vi "test_riccat_01i.vi"() -> (3 "All Tests Passed":bool)   [LabVIEW 2019]
uses:
  <vilib>/Analysis/Matrix/Datatypes/RealMatrix.ctl
  <vilib>/Rock Robotics/WPI/ThirdParty/JAS_Junk/TrajLib/Trajectory_Library.lvlib
  <vilib>/Analysis/Matrix/NI_Matrix.lvlib
panel:
  out "Verify Passed":bool
  out "error out 2":errorcluster
  out "Pos Semi Definite":bool
  out "C":T1
  out "Q_Chk_Passed":bool
  out "Q Check":T1
  out "Stable Bad":bool
  out "Bad":bool
  out "Eigenvalues":cdb[](array[numeric])
  out "error out":errorcluster
  out "Error":bool
  out "Iterations":i32
  out "Elapsed \nTime MS":dbl
  out "ZERO":T1
  out "X  Answer":T1
  in  "R":T1=[[0.25]]
  in  "Q":T1=[[1.0, 0.0, 0.0, 0.0], [0.0, 0.0, 0.0, 0.0], [0.0, 0.0, 0.0, 0.0], [0.0, 0.0, 0.0, 0.0]]
  in  "B":T1=[[0.0], [0.0], [0.0], [1.0]]
  in  "A":T1=[[0.5, 1.0, 0.0, 0.0], [0.0, 0.0, 1.0, 0.0], [0.0, 0.0, 0.0, 1.0], [0.0, 0.0, 0.0, 0.0]]
  # "Test 1: non-invertible A\n  // Example 2 of \"On the Numerical Solution of the Discrete-Time Algebraic\n  // Riccati Equation\""
  # "int n1 = 4, m1 = 1;"
  # "Example = F"
  # "MatrixXd A1(n1, n1), B1(n1, m1), Q1(n1, n1), R1(m1, m1);"
  # "A1 << 0.5, 1, 0, 0, \n          0, 0, 1, 0, \n          0, 0, 0, 1, \n          0, 0, 0, 0;"
  # "B1 << 0, \n        0, \n        0, \n        1;"
  # "Example G1"
  # "Example H"
  # "Solution weight ??"
  # "Q1 << 1, 0, 0, 0, \n        0, 0, 0, 0, \n        0, 0, 0, 0, \n        0, 0, 0, 0;"
  # "Example G2"
  # "Cost ??"
  # "R1 << 0.25;"
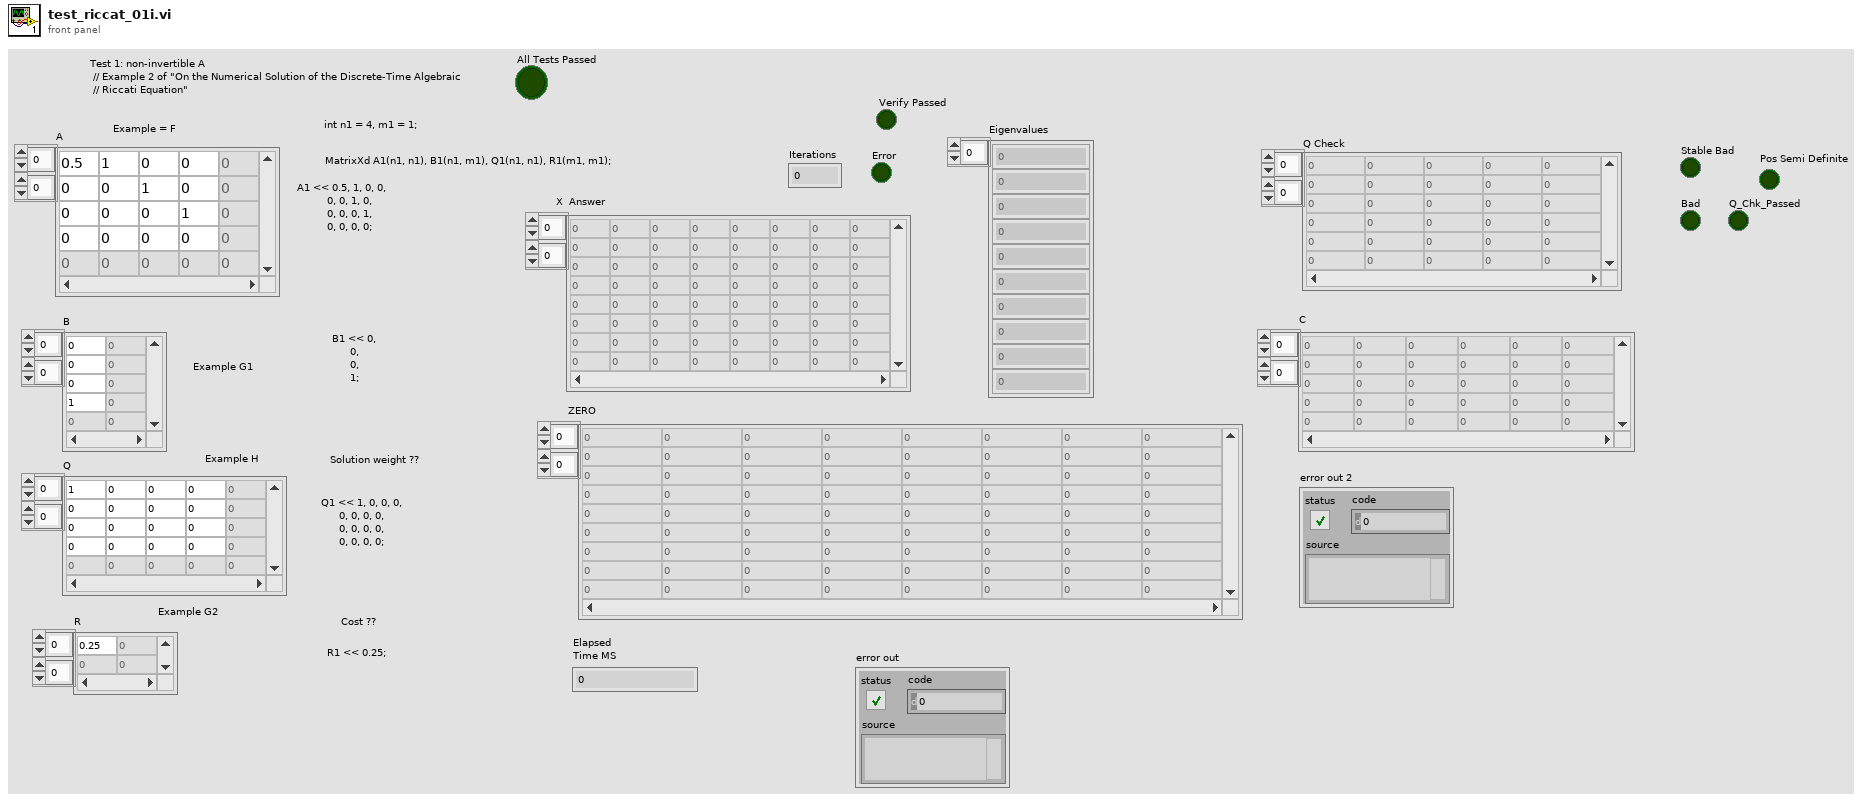
[diagram p1: front panel]
types:
  T1 = typedef "NI_Matrix.lvlib/RealMatrix.ctl" = dbl[][]
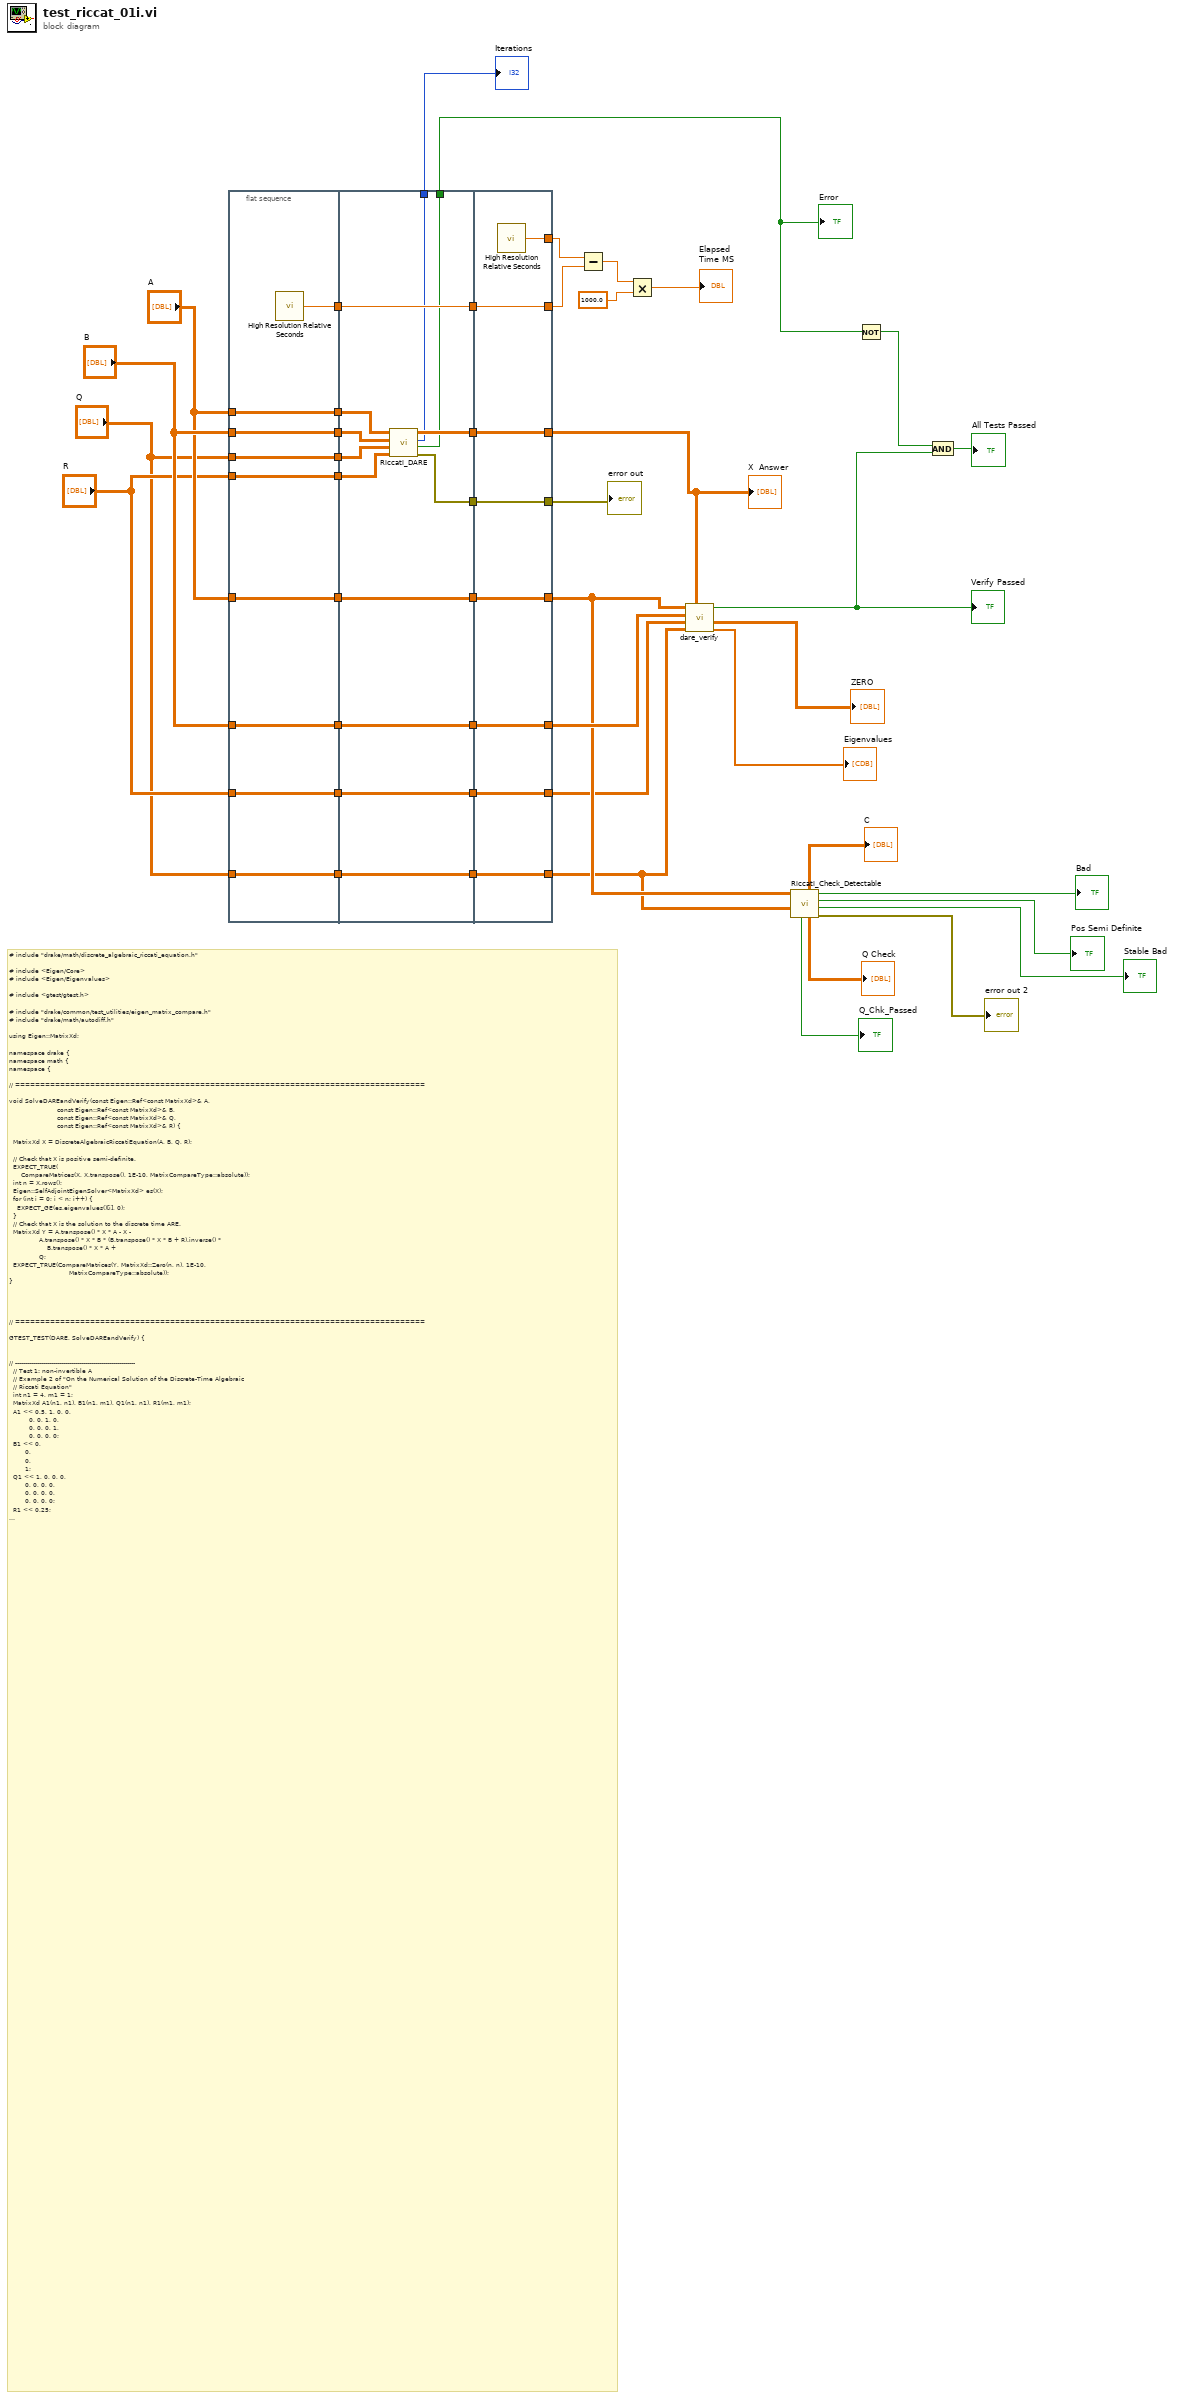
[diagram p0: block diagram]
diagram:
  # "# include \"drake/math/discrete_algebraic_riccati_equation.h\"\n\n# include <Eigen/Core>\n# include <Eigen/Eigenvalues>\n\n# include <gtest/gtest.h>\n\n# include \"drake/common/test_utilities/eigen_matrix_compare.h\"\n# include \"drake/math/autodiff.h\"\n\nusing Eigen::MatrixXd;\n\nnamespace drake {\nnamespace math {\nnamespace {\n\n// ==================================================================================\n\nvoid SolveDAREandVerify(const Eigen::Ref<const MatrixXd>& A,\n                        const Eigen::Ref<const MatrixXd>& B,\n                        const Eigen::Ref<const MatrixXd>& Q,\n                        const Eigen::Ref<const MatrixXd>& R) {\n\n  MatrixXd X = DiscreteAlgebraicRiccatiEquation(A, B, Q, R);\n\n  // Check that X is positive semi-definite.\n  EXPECT_TRUE(\n      CompareMatrices(X, X.transpose(), 1E-10, MatrixCompareType::absolute));\n  int n = X.rows();\n  Eigen::SelfAdjointEigenSolver<MatrixXd> es(X);\n  for (int i = 0; i < n; i++) {\n    EXPECT_GE(es.eigenvalues()[i], 0);\n  }\n  // Check that X is the solution to the discrete time ARE.\n  MatrixXd Y = A.transpose() * X * A - X -\n               A.transpose() * X * B * (B.transpose() * X * B + R).inverse() *\n                   B.transpose() * X * A +\n               Q;\n  EXPECT_TRUE(CompareMatrices(Y, MatrixXd::Zero(n, n), 1E-10,\n                              MatrixCompareType::absolute));\n}\n\n\n\n\n// ==================================================================================\n\nGTEST_TEST(DARE, SolveDAREandVerify) {\n\n\n// ------------------------------------------------------------\n  // Test 1: non-invertible A\n  // Example 2 of \"On the Numerical Solution of the Discrete-Time Algebraic\n  // Riccati Equation\"\n  int n1 = 4, m1 = 1;\n  MatrixXd A1(n1, n1), B1(n1, m1), Q1(n1, n1), R1(m1, m1);\n  A1 << 0.5, 1, 0, 0, \n          0, 0, 1, 0, \n          0, 0, 0, 1, \n          0, 0, 0, 0;\n  B1 << 0, \n        0, \n        0, \n        1;\n  Q1 << 1, 0, 0, 0, \n        0, 0, 0, 0, \n        0, 0, 0, 0, \n        0, 0, 0, 0;\n  R1 << 0.25;\n  SolveDAREandVerify(A1, B1, Q1, R1);\n// ------------------------------------------------------------\n  // Test 2: invertible A\n  int n2 = 2, m2 = 1;\n  MatrixXd A2(n2, n2), B2(n2, m2), Q2(n2, n2), R2(m2, m2);\n  A2 << 1, 1, 0, 1;\n  B2 << 0, 1;\n  Q2 << 1, 0, 0, 0;\n  R2 << 0.3;\n  SolveDAREandVerify(A2, B2, Q2, R2);\n\n// ------------------------------------------------------------\n  // Test 3: the first generalized eigenvalue of (S,T) is stable\n  int n3 = 2, m3 = 1;\n  MatrixXd A3(n3, n3), B3(n3, m3), Q3(n3, n3), R3(m3, m3);\n  A3 << 0, 1, 0, 0;\n  B3 << 0, 1;\n  Q3 << 1, 0, 0, 1;\n  R3 << 1;\n  SolveDAREandVerify(A3, B3, Q3, R3);\n\n// ------------------------------------------------------------\n  // Test 4: A = B = Q = R = I_2 (2-by-2 identity matrix)\n  int n4 = 2, m4 = 2;\n  MatrixXd A4(n4, n4), B4(n4, m4), Q4(n4, n4), R4(m4, m4);\n  A4 << 1, 0, 0, 1;\n  B4 << 1, 0, 0, 1;\n  Q4 << 1, 0, 0, 1;\n  R4 << 1, 0, 0, 1;\n  SolveDAREandVerify(A4, B4, Q4, R4);\n\n// ------------------------------------------------------------\n}\n}  // namespace\n}  // namespace math\n}  // namespace drake"
  n1 = flat-sequence {
    tunnel: "B" -> [w49]
    tunnel: "A" -> [w50]
    tunnel: "B" -> [w51]
    tunnel: "Q" -> [w52]
    tunnel: "A" -> [w53]
    tunnel: "R" -> [w54]
    tunnel: [w54] -> w45
    tunnel: [w53] -> w44
    tunnel: [w52] -> w43
    tunnel: [w51] -> w42
    tunnel: [w50] -> w41
    tunnel: [w49] -> w40
    tunnel: "R" -> [w48]
    tunnel: [w48] -> w33
    tunnel: "Q" -> [w47]
    tunnel: [w47] -> w31
    tunnel: [w46] -> w25
    tunnel: w45 -> [w67]
    tunnel: w44 -> [w65]
    tunnel: w43 -> [w64]
    tunnel: w42 -> [w63]
    tunnel: w41 -> [w62]
    tunnel: w40 -> [w61]
    tunnel: [w66] -> w39
    tunnel: [w62] -> w38
    tunnel: [w61] -> w37
    tunnel: [w60] -> w34
    tunnel: w33 -> [w60]
    tunnel: w31 -> [w59]
    tunnel: [w59] -> w30
    tunnel: [w58] -> w26
    tunnel: w25 -> [w58]
    tunnel: [w57] -> w21
    tunnel: [w56] -> w20
    tunnel: [w55] -> w19
    tunnel: [w73] -> w16
    tunnel: [w74] -> w10
    tunnel: [w75] -> w17
    tunnel: w39 -> [w75]
    tunnel: w38 -> [w74]
    tunnel: w37 -> [w73]
    tunnel: [w72] -> w9
    tunnel: w34 -> [w72]
    tunnel: [w71] -> w7
    tunnel: w30 -> [w71]
    tunnel: [w70] -> w28
    tunnel: [w69] -> w27
    tunnel: w26 -> [w69]
    tunnel: w19 -> [w68]
    tunnel: [w68] -> w18
    frame #0 {
      n2 = call <vilib>:"High Resolution Relative Seconds.vi"() -> ("relative seconds"=w46:dbl)
    }
    frame #1 {
      n3 = call <vilib>:"Riccati_DARE.vi"("R"=w67, "Q"=w64, "B"=w63, "A"=w65) -> ("error out"=w55:errorcluster, "Error"=w56:bool, "Iterations"=w57:i32, "Answer"=w66:T1)  [unwired: 4 in]
    }
    frame #2 {
      n4 = call <vilib>:"High Resolution Relative Seconds.vi"() -> ("relative seconds"=w70:dbl)
    }
  }
  n5 = Subtract(x=w28, y=w27) -> (x-y=w24:dbl)
  n6 = Multiply(x=w24, y=1000.0) -> (x*y=→"Elapsed \nTime MS":dbl)
  n7 = call "dare_verify.vi"("Answer"=w17, "Q"=w7, "R"=w9, "B"=w16, "A"=w10) -> ("Eigenvalues"=→"Eigenvalues":cdb[], "ZERO"=→"ZERO":T1, "Passed"=w12:bool)  [unwired: 4 in]
  "Verify Passed" <- w12
  n8 = call <vilib>:"Riccati_Check_Detectable.vi"("Q"=w7, "A"=w10) -> ("error out"=→"error out 2":errorcluster, "Stable Bad"=→"Stable Bad":bool, "Pos Semi Definite"=→"Pos Semi Definite":bool, "Bad"=→"Bad":bool, "Q_Check"=→"Q Check":T1, "C"=→"C":T1, "Q_Chk_Passed"=→"Q_Chk_Passed":bool)  [unwired: 3 in]
  n9 = Not(x=w20) -> (.not. x?=w13:bool)
  n10 = And(x=w13, y=w12) -> (x .and. y?=→"All Tests Passed":bool)
  "X  Answer" <- w17
  "Iterations" <- w21
  "Error" <- w20
  "error out" <- w18
